vi "Delete User.vi"(8 "error in (no error)":errorcluster, 10 "Credential":T1, 11 "Access in":refnum<class "Access.lvclass">) -> (0 "error out":errorcluster, 3 "Access out":refnum<class "Access.lvclass">)   [LabVIEW 2016, in "Database.lvlib" / "Access.lvclass"]
uses:
  Access.lvclass
  DB/Credential.ctl
  Access.lvclass/Access.ctl
  <vilib>/addons/database/NI_Database_API.lvlib
  User Interface/User Interface.lvlib
  Database.lvlib
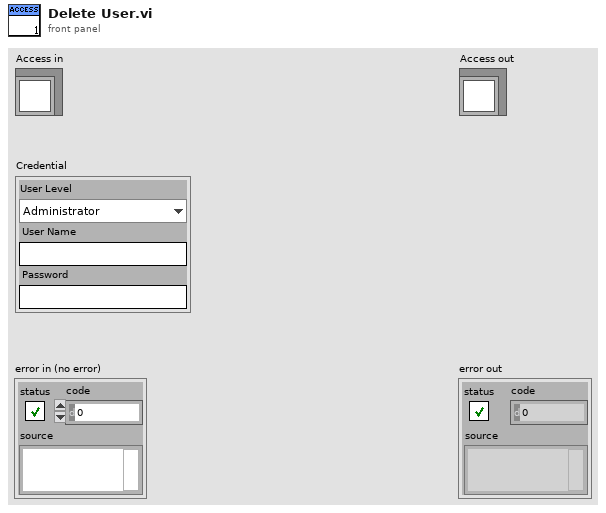
[diagram p1: front panel]
types:
  T1 = typedef "Database.lvlib/Credential.ctl" = cluster{"User Level":enum16{"Administrator", "Engineer", "Operator"}, "User Name":string, "Password":string}
  T2 = typedef "Database.lvlib/DB.lvclass/Table_info.ctl" = cluster{"Authentication":string, "Instr_Configuration":string, "Recipe":string, "Test_data":string}
  T3 = typedef "NI_Database_API.lvlib/Conn ObjectReference.ctl" = refnum<k1>
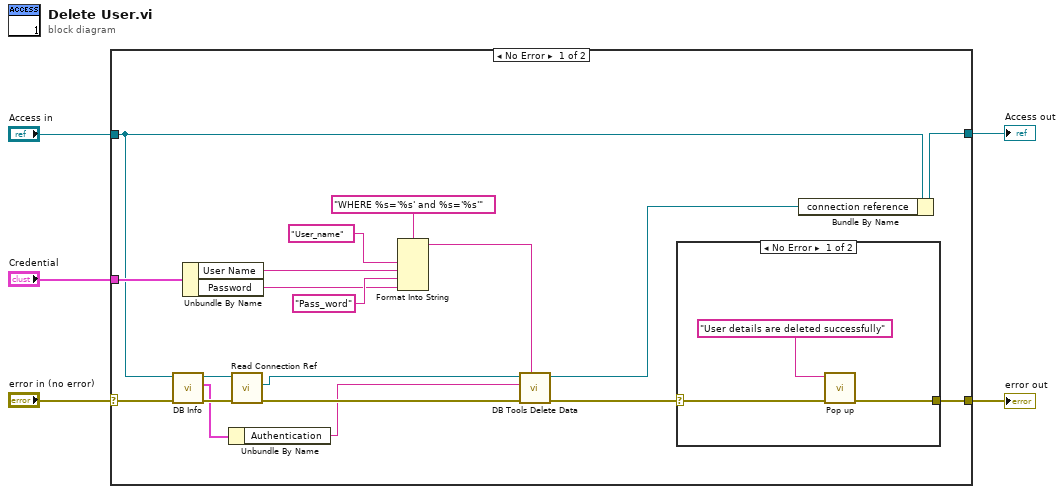
[diagram p0: block diagram]
diagram:
  n1 = case shown="No Error" "error in (no error)" {
    selector: "error in (no error)" -> [w19 w29]
    tunnel: "Access in" -> [w15 w30]
    tunnel: "Credential" -> [w18 _]
    tunnel: [w16 w30] -> w2
    tunnel: [w6 w29] -> w1
    frame No Error {
      n2 = call-dynamic "DB Info.vi"("error in (no error)"=w19, "Access in"=w15) -> ("error out"=w24:errorcluster, "Table_info"=w22:T2, "Access out"=w23:refnum<class "Access.lvclass">)  [unwired: 6 in, 1 out]
      n3 = Unbundle By Name(w18) -> ("User Name"=w14:string, "Password"=w9:string)
      n4 = Unbundle By Name(w22) -> ("Authentication"=w17:string)
      n5 = call-dynamic "Read Connection Ref.vi"("error in (no error)"=w24, "Access in"=w23) -> ("error out"=w21:errorcluster, "connection reference"=w20:T3)  [unwired: 7 in, 1 out]
      n6 = Format Into String(format string="WHERE %s='%s' and %s='%s'" ("condition"), "User_name" ("input 1"), w14, "Pass_word" ("input 3"), w9) -> (resulting string=w11:string)  [unwired: 2 in, 1 out]
      n7 = call <vilib>:"DB Tools Delete Data.vi"("condition"=w11, "error in (no error)"=w21, "table"=w17, "connection reference"=w20) -> ("error out"=w7:errorcluster, "connection reference out"=w8:T3)  [unwired: 6 in]
      n8 = case shown="No Error" w7 {
        selector: w7 -> [w27 w28]
        tunnel: [w26 w28] -> w6
        frame No Error {
          n9 = call "Pop up.vi"("error in (no error)"=w27, "Message In"="User details are deleted successfully") -> ("error out"=w26:errorcluster)  [unwired: 9 in]
        }
        frame Error {
        }
      }
      n10 = Bundle By Name(cluster=w15, "connection reference"=w8) -> (w16:refnum<class "Access.lvclass">)
    }
    frame Error {
    }
  }
  "error out" <- w1
  "Access out" <- w2
